vi "Control.vi"() -> ()   [LabVIEW 2018]
uses:
  <vilib>/Platform/TimedLoop/XDataNode/timing_clust.ctl
  <vilib>/Platform/TimedLoop/XDataNode/nitl_modes.ctl
  <vilib>/Platform/TimedLoop/XDataNode/wakeup.ctl
  <vilib>/myRIO/Instrument Drivers/Onboard IO/AI/typedefs/AI Reference.ctl
  <vilib>/myRIO/Common/Instrument Driver Framework/Utilities/typedefs/myRIO Generic Hardware Reference.ctl
  <vilib>/myRIO/Common/Instrument Driver Framework/Utilities/typedefs/Hardware Version Enum.ctl
  <vilib>/myRIO/Common/Instrument Driver Framework/Utilities/typedefs/myRIO v1.0 Reference.ctl
  <vilib>/myRIO/Common/Instrument Driver Framework/Utilities/typedefs/Generic FPGA Reference.ctl
  <vilib>/myRIO/Common/Instrument Driver Framework/myRIO v1.0/AI/typedefs/AI Channels List.ctl
  <vilib>/myRIO/Common/Instrument Driver Framework/myRIO v1.0/AI/typedefs/AI Channels Enum.ctl
  <vilib>/myRIO/Common/Instrument Driver Framework/Utilities/typedefs/Analog Scaling Constants List.ctl
  <vilib>/myRIO/Common/Instrument Driver Framework/Utilities/typedefs/Analog Scaling Constants.ctl
  <vilib>/userdefined/High Color/nirio_resource_hc.ctl
  <vilib>/myRIO/Instrument Drivers/Onboard IO/AO/typedefs/AO Reference.ctl
  <vilib>/myRIO/Common/Instrument Driver Framework/myRIO v1.0/AO/typedefs/AO Channels List.ctl
  <vilib>/myRIO/Common/Instrument Driver Framework/myRIO v1.0/AO/typedefs/AO Channels Enum.ctl
  <vilib>/myRIO/Common/Instrument Driver Framework/Utilities/vis/Is FPGA Ref Available.vi
  <vilib>/myRIO/Common/Instrument Driver Framework/myRIO v1.0/AI/vis/myRIO v1.1 Open AI.vi
  <vilib>/myRIO/Instrument Drivers/Onboard IO/AI/vis/Read.vi
  <vilib>/myRIO/Common/Instrument Driver Framework/myRIO v1.0/AO/vis/myRIO v1.1 Open AO.vi
  <vilib>/myRIO/Instrument Drivers/Onboard IO/AO/vis/Write.vi
  <vilib>/myRIO/Common/Instrument Driver Framework/Utilities/vis/Validate Channels.vi
  <vilib>/myRIO/Common/Instrument Driver Framework/myRIO v1.0/AI/vis/myRIO v1.0 Reserve AI.vi
  <vilib>/myRIO/Common/Instrument Driver Framework/myRIO v1.0/AO/vis/myRIO v1.0 Reserve AO.vi
  <vilib>/myRIO/Common/Instrument Driver Framework/myRIO v1.0/AI/vis/myRIO v1.0 Build MUX Configuration AI.vi
  <vilib>/myRIO/Common/Instrument Driver Framework/myRIO v1.0/Resource Manager/vis/myRIO v1.0 Reserve Channel List.vi
  <vilib>/myRIO/Common/Instrument Driver Framework/myRIO v1.0/AO/vis/myRIO v1.0 Build MUX Configuration AO.vi
  <vilib>/myRIO/Common/Instrument Driver Framework/myRIO v1.0/Resource Manager/vis/myRIO v1.0 Reserve Channel.vi
  <vilib>/myRIO/Common/Instrument Driver Framework/myRIO v1.0/Resource Manager/vis/myRIO v1.0 Unreserve Channel.vi
  <vilib>/myRIO/Common/Instrument Driver Framework/myRIO v1.0/Resource Manager/vis/myRIO v1.0 Build Mutex Name.vi
  <vilib>/Utility/VariantDataType/GetNumericInfo.vi
  <vilib>/Utility/error.llb/Error Cluster From Error Code.vi
  <vilib>/myRIO/Common/Instrument Driver Framework/myRIO v1.0/myRIO v1.1 Open.vi
  <vilib>/myRIO/Common/Instrument Driver Framework/myRIO v1.0/AI/vis/myRIO v1.0 Get Scaling Constants AI.vi
  <vilib>/myRIO/Common/Instrument Driver Framework/Utilities/vis/IO Manager.vi
  <vilib>/myRIO/Common/Instrument Driver Framework/Utilities/vis/Configuration Manager.vi
  <vilib>/myRIO/Common/Instrument Driver Framework/myRIO v1.0/myRIO v1.0 Close.vi
  <vilib>/myRIO/Common/Instrument Driver Framework/myRIO v1.0/AI/vis/myRIO v1.0 Read AI.vi
  <vilib>/myRIO/Common/Instrument Driver Framework/myRIO v1.0/AO/vis/myRIO v1.0 Get Scaling Constants AO.vi
  <vilib>/myRIO/Common/Instrument Driver Framework/myRIO v1.0/AO/vis/myRIO v1.0 Write AO.vi
  <vilib>/platform/TimedLoop/XDataNode/XDataNode.xnode
  <vilib>/myRIO/Express VI/Onboard IO/AI/AI Express VI.xnode
  <vilib>/myRIO/Instrument Drivers/Onboard IO/AI/vis/myRIO AI Open.xnode
  <vilib>/myRIO/Express VI/Onboard IO/AO/AO Express VI.xnode
  <vilib>/myRIO/Instrument Drivers/Onboard IO/AO/vis/myRIO AO Open.xnode
  <vilib>/myRIO/Instrument Drivers/Onboard IO/AI/AI.lvlib
  <vilib>/myRIO/Instrument Drivers/Onboard IO/AO/AO.lvlib
  <vilib>/Platform/TimedLoop/XDataNode/XDNodeRunTimeDep.lvlib
panel:
  in  "Operating Mode":string(combo)="1"
  in  "Upper Bound":dbl=0.1 format="%#_13g"
  in  "Lower Bound":dbl=0.04 format="%#_13g"
  in  "Signal Frequency / Hz":i64=200
  in  "Factor of Decrease":dbl=1e-05
  in  "Factor of Increase":dbl=1e-05
  out "SoVal":bool
  in  "SELF-DESTRUCT BUTTON":bool
  out "BIGGER SELF-DESTRUCT BUTTON":bool
  out "SoVal\nSoVal (C/AO0 (AO0))":dbl
  out "Gas Reg. (A/AO0 (Pin 2))":dbl=0.04 min=0.04 max=0.1
  in  "Setpoint":dbl=5.5
  out "Force Resistor":dbl
  out "FSR 2":dbl(knob) scale=-9.0..11.0
  out "PP 2":dbl
  out "PRESSURE PAD":dbl(knob) scale=-11.0..11.0
  out "PP":bool
  out "FSR":bool
  in  "PP Weight":dbl=0.001 min=0.0 max=1.0 step=0.001
  in  "FSR Weight":dbl=0.1 min=0.0 max=1.0 step=0.0001
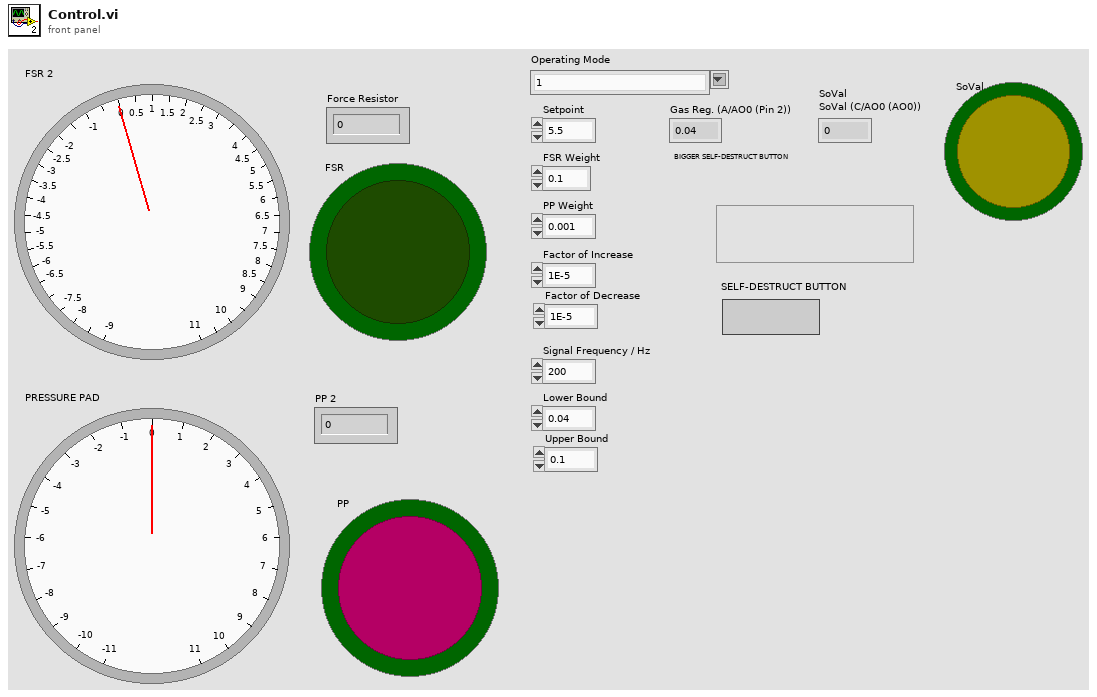
[diagram p1: front panel]
types:
  T1 = typedef "XDNodeRunTimeDep.lvlib/timing_clust.ctl" = cluster{"Expected End [f-1]":u64, "Actual End [f-1]":u64, "Finished Late? [f-1]":bool, "Expected End [i-1]":u64, "Actual End [i-1]":u64, "Finished Late? [i-1]":bool, "Expected Start [i]":u64, "Actual Start [i]":u64, "Expected Start [f]":u64, "Actual Start [f]":u64, "Source Name":string, "Structure Name":string, "Period":i64, "Deadline":i64, "Offset":i64, "Start":i64, "Priority":i32, "Timeout":i32, "Mode":T2, "Wakeup Reason":T3, "Error":errorcluster, "Source Type":string, "Secondary Source Type":string, "Global End Time":u64, "Global Start Time":u64, "Frame Duration":u64, "Iteration Duration":u64, "Assigned CPU":i32, "I/O Scan Engine Mode":u32}
  T2 = typedef "XDNodeRunTimeDep.lvlib/nitl_modes.ctl" = enum32{"No Change", "Process missed periods, maintain original phase", "Discard missed periods, maintain original phase", "Process missed periods, ignore original phase", "Discard missed periods, ignore original phase"}
  T3 = typedef "XDNodeRunTimeDep.lvlib/wakeup.ctl" = enum32{"Normal", "Aborted", "Asynchronous wakeup", "Timing source error", "Timed loop error", "Timeout"}
  T4 = typedef "AO.lvlib/AO Reference.ctl" = cluster{"myRIO Reference":T5, "AO Channel List":T9, "AO Scaling Constant List":T11}
  T5 = typedef "myRIO Generic Hardware Reference.ctl" = cluster{"myRIO Model":T6, "myRIO Hardware Reference":T7}
  T6 = typedef "Hardware Version Enum.ctl" = enum16{"Unknown", "myRIO-1900", "myRIO-1950", "roboRIO", "NI ELVIS RIO CM", "ELVIS III"}
  T7 = typedef "myRIO v1.0 Reference.ctl" = cluster{"Generic FPGA Reference":T8, "Allow multiple opens":bool}
  T8 = typedef "Generic FPGA Reference.ctl" = refnum<k20>
  T9 = typedef "AO Channels List.ctl" = T10[]
  T10 = typedef "AO Channels Enum.ctl" = enum16{"Not Connected", "AudioOut/Left", "AudioOut/Right", "C/AO0", "C/AO1", "A/AO0", "A/AO1", "B/AO0", "B/AO1"}
  T11 = typedef "Analog Scaling Constants List.ctl" = T12[]
  T12 = typedef "Analog Scaling Constants.ctl" = cluster{"LSB Weight (Volts)":dbl, "Offset (Volts)":dbl, "Signed?":bool}
  T13 = typedef "nirio_resource_hc.ctl" = tag
  T14 = typedef "AI.lvlib/AI Reference.ctl" = cluster{"myRIO Reference":T5, "AI Channels List":T15, "AI Scaling Constants List":T11}
  T15 = typedef "AI Channels List.ctl" = T16[]
  T16 = typedef "AI Channels Enum.ctl" = enum16{"Not Connected", "AudioIn/Left", "AudioIn/Right", "C/AI0", "C/AI1", "A/AI0", "A/AI1", "A/AI2", "A/AI3", "A/AI4", "A/AI5", "A/AI6", "A/AI7", "B/AI0", "B/AI1", "B/AI2", "B/AI3", "B/AI4", "B/AI5", "B/AI6", "B/AI7", "AI/AI0", "AI/AI1", "AI/AI2", "AI/AI3", "A/AI0 (DIFF)", "A/AI1 (DIFF)", "A/AI2 (DIFF)", "A/AI3 (DIFF)", "B/AI0 (DIFF)", "B/AI1 (DIFF)", "B/AI2 (DIFF)", "B/AI3 (DIFF)"}
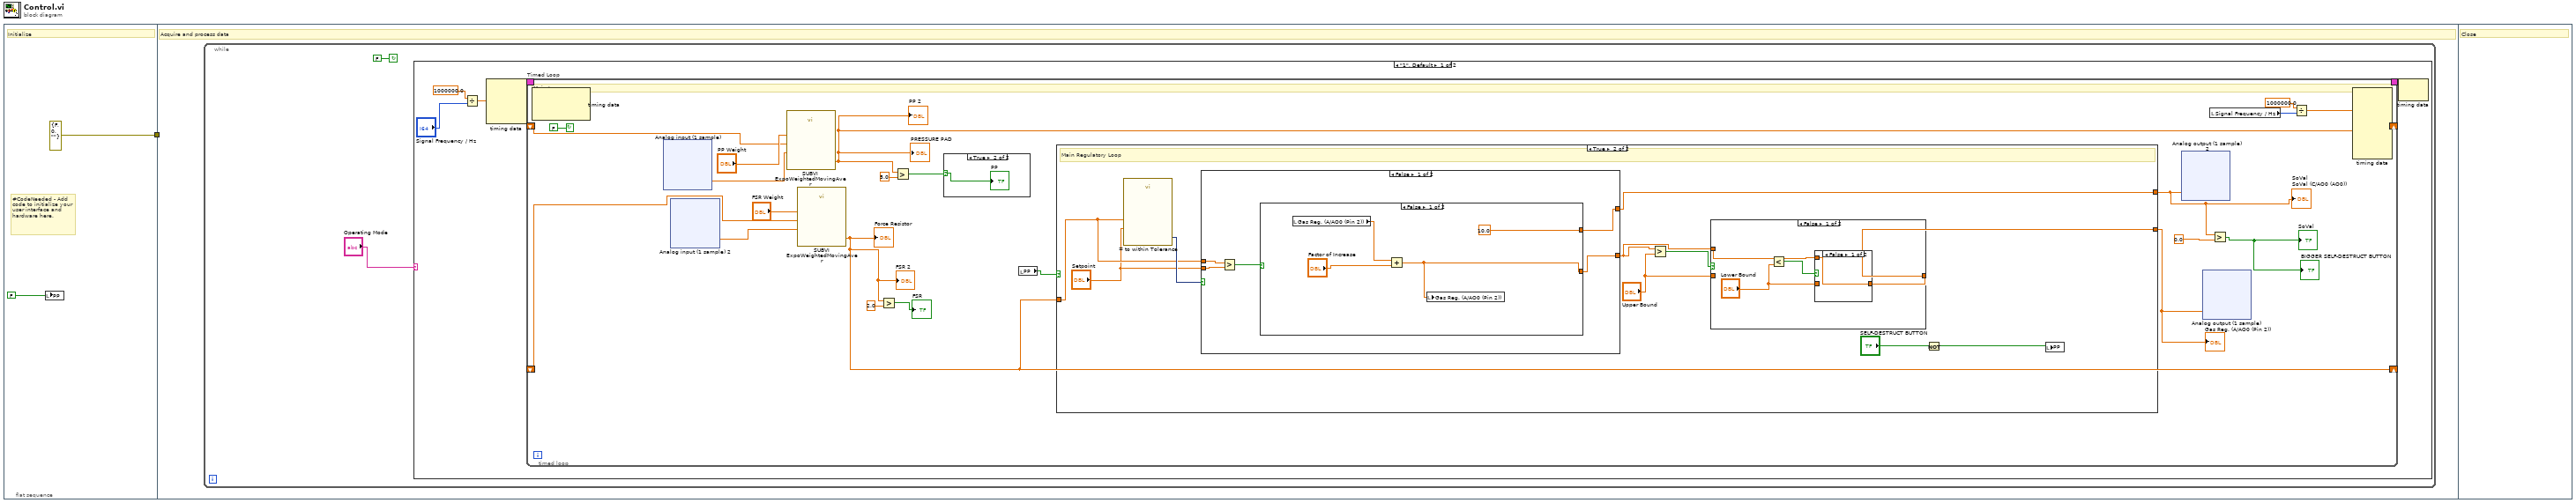
[diagram p0: block diagram]
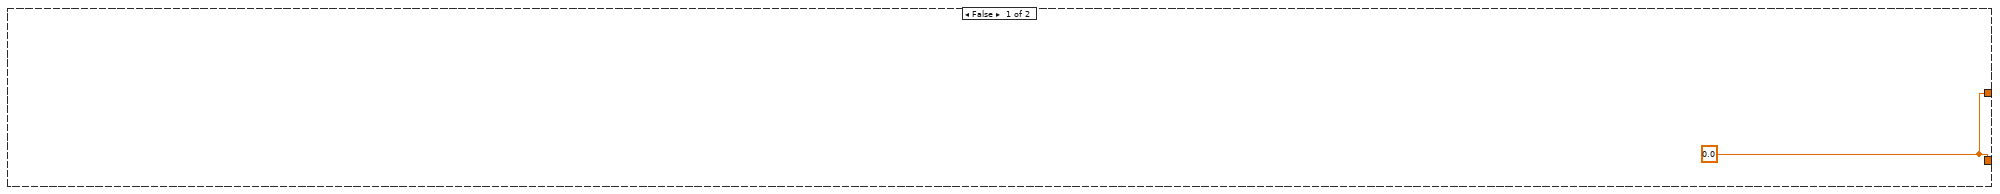
[diagram p2: hidden frame]
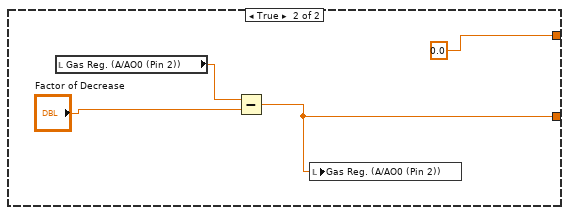
[diagram p5: hidden frame]
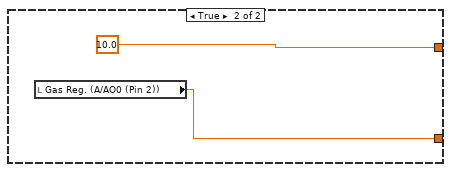
[diagram p6: hidden frame]
diagram:
  n1 = flat-sequence {
    tunnel: [errorcluster {"status"=FALSE, "code"=0, "source"=""} ("error in (no error)")] -> w1
    tunnel: w1 -> [_]
    frame #0 {
      # "#CodeNeeded - Add code to initialize your user interface and hardware here."
      # "Initialize"
      n2 = local write "PP"(FALSE ("PP")) -> ()
    }
    frame #1 {
      # "Acquire and process data"
      n3 = while {
        stop <- FALSE continue-if-true
        n4 = case shown="\"1\", Default" "Operating Mode" {
          frame "1", Default {
            n5 = Divide(x=1000000.0, y="Signal Frequency / Hz") -> (x/y=w8:dbl)
            n6 = node-c288(w8) -> (w10:T1)  [unwired: 3 in]
            n7 = timed-loop "Timed Loop" {
              shift-right: [w24] -> _
              shift-left: _ -> [w26]
              shift-right: [w18] -> _
              shift-left: _ -> [w22]
              timing: w10 -> [_]
              timing-out: [_] -> w9
              stop <- FALSE continue-if-true
              # "Main Loop"
              n8 = node-c288() -> ()  [unwired: 1 in, 3 out]
              n9 = xnode "Analog input (1 sample)"() -> ("PP (C/AI1 (AI1))"=w25:dbl)  [unwired: 1 in, 1 out]
              n10 = xnode "Analog input (1 sample) 2"() -> ("FSR (C/AI0 (AI0))"=w23:dbl)  [unwired: 1 in, 1 out]
              n11 = call "SUBVI ExpoWeightedMovingAver.vi"("New Sample"=w25, "EWMA Weight"="PP Weight", "Old Estimate"=w26) -> ("Weighted Average"=w24:dbl)  [unwired: 8 in]
              "PP 2" <- w24
              "PRESSURE PAD" <- w24
              n12 = call "SUBVI ExpoWeightedMovingAver.vi"("New Sample"=w23, "EWMA Weight"="FSR Weight", "Old Estimate"=w22) -> ("Weighted Average"=w18:dbl)  [unwired: 8 in]
              "Force Resistor" <- w18
              "FSR 2" <- w18
              n13 = Greater?(x=w18, y=2.0) -> (0:→"FSR":bool)
              n14 = Greater?(x=w24, y=5.0) -> (0:w20:bool)
              n15 = case shown="True" w20 {
                selector: w20 -> [_ w143]
                frame False {
                }
                frame True {
                  "PP" <- w143
                }
              }
              n16 = local read "PP"() -> (w19:bool)
              n17 = case shown="True" w19 {
                tunnel: w18 -> [_ w119]
                tunnel: [w110 w114] -> w17
                tunnel: [w110 w113] -> w16
                frame False {
                  w110 = 0.0
                }
                frame True {
                  # "Main Regulatory Loop"
                  n18 = call "= to within Tolerance"("Constant Value to Compare Against"="Setpoint", "Operand 1"=w119) -> ("Result"=w120:dynamicdata)  [unwired: 8 in, 1 out]
                  n19 = case shown="False" w120 {
                    tunnel: [w129 w142] -> w116
                    tunnel: w119 -> [w132 _]
                    tunnel: "Setpoint" -> [w131 _]
                    tunnel: [w128 10.0 ("SoVal\nSoVal (C/AO0 (AO0))")] -> w113
                    frame False {
                      n20 = Greater?(x=w132, y=w131) -> (0:w130:bool)
                      n21 = case shown="False" w130 {
                        tunnel: [w136 w139] -> w129
                        tunnel: [10.0 0.0] -> w128
                        frame False {
                          n22 = local read "Gas Reg. (A/AO0 (Pin 2))"() -> (w135:dbl)
                          n23 = Add(x=w135, y="Factor of Increase") -> (x+y=w136:dbl)
                          n24 = local write "Gas Reg. (A/AO0 (Pin 2))"(w136) -> ()
                        }
                        frame True {
                          n25 = local read "Gas Reg. (A/AO0 (Pin 2))"() -> (w140:dbl)
                          n26 = Subtract(x=w140, y="Factor of Decrease") -> (x-y=w139:dbl)
                          n27 = local write "Gas Reg. (A/AO0 (Pin 2))"(w139) -> ()
                        }
                      }
                    }
                    frame True {
                      n28 = local read "Gas Reg. (A/AO0 (Pin 2))"() -> (w142:dbl)
                    }
                  }
                  n29 = Greater?(x=w116, y="Upper Bound") -> (0:w117:bool)
                  n30 = case shown="False" w117 {
                    tunnel: w116 -> [w121 _]
                    tunnel: [w122 w127] -> w114
                    tunnel: "Upper Bound" -> [_ w127]
                    frame False {
                      n31 = Less?(x=w121, y="Lower Bound") -> (x < y?=w124:bool)
                      n32 = case shown="False" w124 {
                        tunnel: [w125 w126] -> w122
                        tunnel: "Lower Bound" -> [_ w126]
                        tunnel: w121 -> [w125 _]
                        frame False {
                        }
                        frame True {
                        }
                      }
                    }
                    frame True {
                    }
                  }
                  n33 = Not(x="SELF-DESTRUCT BUTTON") -> (.not. x?=w111:bool)
                  n34 = local write "PP"(w111) -> ()
                }
              }
              "Gas Reg. (A/AO0 (Pin 2))" <- w17
              "SoVal\nSoVal (C/AO0 (AO0))" <- w16
              n35 = xnode "Analog output (1 sample) 2"("C/AO0 (AO0)"=w16) -> ()  [unwired: 1 in, 1 out]
              n36 = xnode "Analog output (1 sample)"("Gas Reg. (A/AO0 (Pin 2))"=w17) -> ()  [unwired: 1 in, 1 out]
              n37 = local read "Signal Frequency / Hz"() -> (w12:i64)
              n38 = Greater?(x=w16, y=0.0) -> (0:→"SoVal" →"BIGGER SELF-DESTRUCT BUTTON":bool)
              n39 = Divide(x=1000000.0, y=w12) -> (x/y=w11:dbl)
              n40 = node-c288(w11) -> ()  [unwired: 7 in, 1 out]
            }
            n41 = node-c288(w9) -> ()  [unwired: 1 out]
          }
          frame "2" {
          }
        }
      }
    }
    frame #2 {
      # "Close"
    }
  }
